vi "TestMacroEngineALB.vi"   [LabVIEW 2017]
types:
  T1 = typedef "MacrosALB.ctl" = cluster{"MacroName":string, "Sequence":cluster{"Buttons 1":T2, "Axes 1":T3, "Buttons 2":T4, "Axes 2":T5, "Delay":u32}[], "TotalTime":u32}
  T2 = typedef "JoyStick1ALB.ctl" = cluster{"J1-B0":bool, "J1-B1":bool, "J1-B2":bool, "J1-B3":bool, "J1-B4":bool, "J1-B5":bool, "J1-B6":bool, "J1-B7":bool, "J1-B8-":bool, "J1-B9":bool, "J1-B10":bool, "J1-B11":bool}
  T3 = typedef "JoyStick1ALV(Analog).ctl" = cluster{"Axis 0":dbl, "Axis 1":dbl, "Axis 2":dbl, "Slider":dbl}
  T4 = typedef "JoyStick2ALB.ctl" = cluster{"J2-B0":bool, "J2-B1":bool, "J2-B2":bool, "J2-B3":bool, "J2-B4":bool, "J2-B5":bool, "J2-B6":bool, "J2-B7":bool, "J2-B8":bool, "J2-B9":bool, "J2-B10":bool, "J2-B11":bool}
  T5 = typedef "JoyStick2ALB(Analog).ctl" = cluster{"Axis 0":dbl, "Axis 1":dbl, "Axis 2":dbl, "Switch":dbl}
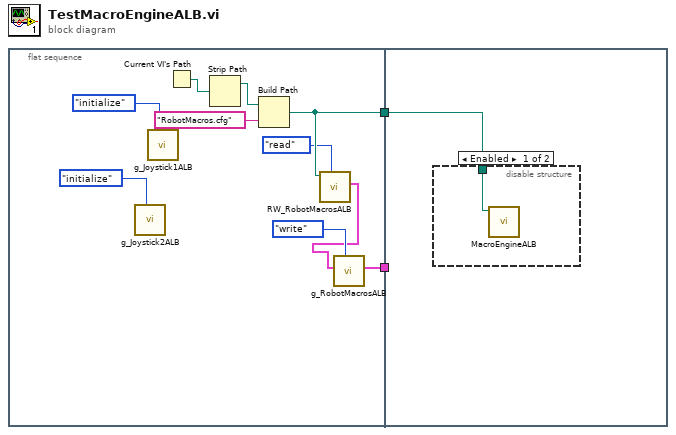
[diagram p0: block diagram]
diagram:
  n1 = flat-sequence {
    tunnel: [w7] -> w2
    tunnel: [w3] -> w1
    tunnel: w2 -> [w13]
    tunnel: w1 -> [_]
    frame #0 {
      n2 = call "g_Joystick2ALB.vi"("Action"=enum16{"initialize", "read", "write"}."initialize") -> ()  [unwired: 7 in, 4 out]
      n3 = call "g_Joystick1ALB.vi"("Action"=enum16{"initialize", "read", "write"}."initialize") -> ()  [unwired: 7 in, 4 out]
      n4 = Current VI's Path() -> (path=w8:path)
      n5 = Strip Path(path=w8) -> (stripped path=w9:path)  [unwired: 1 out]
      n6 = Build Path(base path=w9, name or relative path="RobotMacros.cfg") -> (appended path=w7:path)
      n7 = call "RW_RobotMacrosALB.vi"("Action"=enum16{"read", "write"}."read", "File Path"=w7) -> ("Macros out"=w4:T1[])  [unwired: 8 in, 1 out]
      n8 = call "g_RobotMacrosALB.vi"("Action"=enum16{"read", "write"}."write", "Macros"=w4) -> ("Macros out"=w3:T1[])  [unwired: 9 in]
    }
    frame #1 {
      n9 = disable-structure shown="Enabled" {
        disable-tunnel: w13 -> [w14 _]
        frame Enabled {
          n10 = call "MacroEngineALB.vi"("File Path"=w14) -> ()  [unwired: 11 in]
        }
        frame Disabled {
        }
      }
    }
  }
